vi "读取校准数据.vi"(8 "error in (no error)":errorcluster) -> (0 "error out":errorcluster)   [LabVIEW 2016, in "斯坦道通用流路CODmn.lvlib"]
uses:
  <vilib>/Utility/config.llb/NI_LVConfig.lvlib
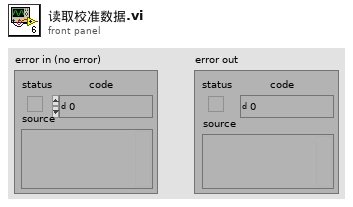
[diagram p1: front panel]
types:
  T1 = cluster{"参数":cluster{"String":string, "Value":u16}, "曲线模型":cluster{"标液浓度1":dbl, "测量吸光度1":dbl, "样品1启用":bool, "标液浓度2":dbl, "测量吸光度2":dbl, "样品2启用":bool, "标液浓度3":dbl, "测量吸光度3":dbl, "样品3启用":bool, "标液浓度4":dbl, "测量吸光度4":dbl, "样品4启用":bool, "标液浓度5":dbl, "测量吸光度5":dbl, "样品5启用":bool, "模型":enum32{"线性", "多项式"}, "精度":dbl, "XY图":cluster{"X Values":dbl[], "Y Values":dbl[]}[], "拟合公式":string, "r^2":dbl, "标样一校准时间":timestamp, "标样二校准时间":timestamp, "标样三校准时间":timestamp, "标样四校准时间":timestamp, "标样五校准时间":timestamp, "方程":cluster{"c":dbl, "x":dbl, "x^2":dbl}, "标定时间":timestamp}[]}[]
  T2 = cluster{"标液浓度1":dbl, "测量吸光度1":dbl, "样品1启用":bool, "标液浓度2":dbl, "测量吸光度2":dbl, "样品2启用":bool, "标液浓度3":dbl, "测量吸光度3":dbl, "样品3启用":bool, "标液浓度4":dbl, "测量吸光度4":dbl, "样品4启用":bool, "标液浓度5":dbl, "测量吸光度5":dbl, "样品5启用":bool, "模型":enum32{"线性", "多项式"}, "精度":dbl, "XY图":cluster{"X Values":dbl[], "Y Values":dbl[]}[], "拟合公式":string, "r^2":dbl, "标样一校准时间":timestamp, "标样二校准时间":timestamp, "标样三校准时间":timestamp, "标样四校准时间":timestamp, "标样五校准时间":timestamp, "二次方程":cluster{"c":dbl, "x":dbl, "x^2":dbl}, "标定时间":timestamp}[]
  T3 = cluster{cluster{"String":string, "Value":u16}, "总磷曲线模型":cluster{"标液浓度1":dbl, "测量吸光度1":dbl, "样品1启用":bool, "标液浓度2":dbl, "测量吸光度2":dbl, "样品2启用":bool, "标液浓度3":dbl, "测量吸光度3":dbl, "样品3启用":bool, "标液浓度4":dbl, "测量吸光度4":dbl, "样品4启用":bool, "标液浓度5":dbl, "测量吸光度5":dbl, "样品5启用":bool, "模型":enum32{"线性", "多项式"}, "精度":dbl, "XY图":cluster{"X Values":dbl[], "Y Values":dbl[]}[], "拟合公式":string, "r^2":dbl, "标样一校准时间":timestamp, "标样二校准时间":timestamp, "标样三校准时间":timestamp, "标样四校准时间":timestamp, "标样五校准时间":timestamp, "二次方程":cluster{"c":dbl, "x":dbl, "x^2":dbl}, "标定时间":timestamp}[]}
  T4 = cluster{cluster{"String":string, "Value":u16}, "总氮曲线模型":cluster{"标液浓度1":dbl, "测量吸光度1":dbl, "样品1启用":bool, "标液浓度2":dbl, "测量吸光度2":dbl, "样品2启用":bool, "标液浓度3":dbl, "测量吸光度3":dbl, "样品3启用":bool, "标液浓度4":dbl, "测量吸光度4":dbl, "样品4启用":bool, "标液浓度5":dbl, "测量吸光度5":dbl, "样品5启用":bool, "模型":enum32{"线性", "多项式"}, "精度":dbl, "XY图":cluster{"X Values":dbl[], "Y Values":dbl[]}[], "拟合公式":string, "r^2":dbl, "标样一校准时间":timestamp, "标样二校准时间":timestamp, "标样三校准时间":timestamp, "标样四校准时间":timestamp, "标样五校准时间":timestamp, "二次方程":cluster{"c":dbl, "x":dbl, "x^2":dbl}, "标定时间":timestamp}[]}
  T5 = cluster{cluster{"String":string, "Value":u16}, "氨氮曲线模型":cluster{"标液浓度1":dbl, "测量吸光度1":dbl, "样品1启用":bool, "标液浓度2":dbl, "测量吸光度2":dbl, "样品2启用":bool, "标液浓度3":dbl, "测量吸光度3":dbl, "样品3启用":bool, "标液浓度4":dbl, "测量吸光度4":dbl, "样品4启用":bool, "标液浓度5":dbl, "测量吸光度5":dbl, "样品5启用":bool, "模型":enum32{"线性", "多项式"}, "精度":dbl, "XY图":cluster{"X Values":dbl[], "Y Values":dbl[]}[], "拟合公式":string, "r^2":dbl, "标样一校准时间":timestamp, "标样二校准时间":timestamp, "标样三校准时间":timestamp, "标样四校准时间":timestamp, "标样五校准时间":timestamp, "二次方程":cluster{"c":dbl, "x":dbl, "x^2":dbl}, "标定时间":timestamp}[]}
  T6 = cluster{cluster{"String":string, "Value":u16}, "磷酸盐曲线模型":cluster{"标液浓度1":dbl, "测量吸光度1":dbl, "样品1启用":bool, "标液浓度2":dbl, "测量吸光度2":dbl, "样品2启用":bool, "标液浓度3":dbl, "测量吸光度3":dbl, "样品3启用":bool, "标液浓度4":dbl, "测量吸光度4":dbl, "样品4启用":bool, "标液浓度5":dbl, "测量吸光度5":dbl, "样品5启用":bool, "模型":enum32{"线性", "多项式"}, "精度":dbl, "XY图":cluster{"X Values":dbl[], "Y Values":dbl[]}[], "拟合公式":string, "r^2":dbl, "标样一校准时间":timestamp, "标样二校准时间":timestamp, "标样三校准时间":timestamp, "标样四校准时间":timestamp, "标样五校准时间":timestamp, "二次方程":cluster{"c":dbl, "x":dbl, "x^2":dbl}, "标定时间":timestamp}[]}
  T7 = cluster{cluster{"String":string, "Value":u16}, "硝氮曲线模型":cluster{"标液浓度1":dbl, "测量吸光度1":dbl, "样品1启用":bool, "标液浓度2":dbl, "测量吸光度2":dbl, "样品2启用":bool, "标液浓度3":dbl, "测量吸光度3":dbl, "样品3启用":bool, "标液浓度4":dbl, "测量吸光度4":dbl, "样品4启用":bool, "标液浓度5":dbl, "测量吸光度5":dbl, "样品5启用":bool, "模型":enum32{"线性", "多项式"}, "精度":dbl, "XY图":cluster{"X Values":dbl[], "Y Values":dbl[]}[], "拟合公式":string, "r^2":dbl, "标样一校准时间":timestamp, "标样二校准时间":timestamp, "标样三校准时间":timestamp, "标样四校准时间":timestamp, "标样五校准时间":timestamp, "二次方程":cluster{"c":dbl, "x":dbl, "x^2":dbl}, "标定时间":timestamp}[]}
  T8 = cluster{cluster{"String":string, "Value":u16}, "亚硝氮曲线模型":cluster{"标液浓度1":dbl, "测量吸光度1":dbl, "样品1启用":bool, "标液浓度2":dbl, "测量吸光度2":dbl, "样品2启用":bool, "标液浓度3":dbl, "测量吸光度3":dbl, "样品3启用":bool, "标液浓度4":dbl, "测量吸光度4":dbl, "样品4启用":bool, "标液浓度5":dbl, "测量吸光度5":dbl, "样品5启用":bool, "模型":enum32{"线性", "多项式"}, "精度":dbl, "XY图":cluster{"X Values":dbl[], "Y Values":dbl[]}[], "拟合公式":string, "r^2":dbl, "标样一校准时间":timestamp, "标样二校准时间":timestamp, "标样三校准时间":timestamp, "标样四校准时间":timestamp, "标样五校准时间":timestamp, "二次方程":cluster{"c":dbl, "x":dbl, "x^2":dbl}, "标定时间":timestamp}[]}
  T9 = cluster{cluster{"String":string, "Value":u16}, "硅酸盐曲线模型":cluster{"标液浓度1":dbl, "测量吸光度1":dbl, "样品1启用":bool, "标液浓度2":dbl, "测量吸光度2":dbl, "样品2启用":bool, "标液浓度3":dbl, "测量吸光度3":dbl, "样品3启用":bool, "标液浓度4":dbl, "测量吸光度4":dbl, "样品4启用":bool, "标液浓度5":dbl, "测量吸光度5":dbl, "样品5启用":bool, "模型":enum32{"线性", "多项式"}, "精度":dbl, "XY图":cluster{"X Values":dbl[], "Y Values":dbl[]}[], "拟合公式":string, "r^2":dbl, "标样一校准时间":timestamp, "标样二校准时间":timestamp, "标样三校准时间":timestamp, "标样四校准时间":timestamp, "标样五校准时间":timestamp, "二次方程":cluster{"c":dbl, "x":dbl, "x^2":dbl}, "标定时间":timestamp}[]}
  T10 = cluster{cluster{"String":string, "Value":u16}, "硫化物曲线模型":cluster{"标液浓度1":dbl, "测量吸光度1":dbl, "样品1启用":bool, "标液浓度2":dbl, "测量吸光度2":dbl, "样品2启用":bool, "标液浓度3":dbl, "测量吸光度3":dbl, "样品3启用":bool, "标液浓度4":dbl, "测量吸光度4":dbl, "样品4启用":bool, "标液浓度5":dbl, "测量吸光度5":dbl, "样品5启用":bool, "模型":enum32{"线性", "多项式"}, "精度":dbl, "XY图":cluster{"X Values":dbl[], "Y Values":dbl[]}[], "拟合公式":string, "r^2":dbl, "标样一校准时间":timestamp, "标样二校准时间":timestamp, "标样三校准时间":timestamp, "标样四校准时间":timestamp, "标样五校准时间":timestamp, "二次方程":cluster{"c":dbl, "x":dbl, "x^2":dbl}, "标定时间":timestamp}[]}
  T11 = cluster{cluster{"String":string, "Value":u16}, "CODcr曲线模型":cluster{"标液浓度1":dbl, "测量吸光度1":dbl, "样品1启用":bool, "标液浓度2":dbl, "测量吸光度2":dbl, "样品2启用":bool, "标液浓度3":dbl, "测量吸光度3":dbl, "样品3启用":bool, "标液浓度4":dbl, "测量吸光度4":dbl, "样品4启用":bool, "标液浓度5":dbl, "测量吸光度5":dbl, "样品5启用":bool, "模型":enum32{"线性", "多项式"}, "精度":dbl, "XY图":cluster{"X Values":dbl[], "Y Values":dbl[]}[], "拟合公式":string, "r^2":dbl, "标样一校准时间":timestamp, "标样二校准时间":timestamp, "标样三校准时间":timestamp, "标样四校准时间":timestamp, "标样五校准时间":timestamp, "二次方程":cluster{"c":dbl, "x":dbl, "x^2":dbl}, "标定时间":timestamp}[]}
  T12 = cluster{cluster{"String":string, "Value":u16}, "CODMn曲线模型":cluster{"标液浓度1":dbl, "测量吸光度1":dbl, "样品1启用":bool, "标液浓度2":dbl, "测量吸光度2":dbl, "样品2启用":bool, "标液浓度3":dbl, "测量吸光度3":dbl, "样品3启用":bool, "标液浓度4":dbl, "测量吸光度4":dbl, "样品4启用":bool, "标液浓度5":dbl, "测量吸光度5":dbl, "样品5启用":bool, "模型":enum32{"线性", "多项式"}, "精度":dbl, "XY图":cluster{"X Values":dbl[], "Y Values":dbl[]}[], "拟合公式":string, "r^2":dbl, "标样一校准时间":timestamp, "标样二校准时间":timestamp, "标样三校准时间":timestamp, "标样四校准时间":timestamp, "标样五校准时间":timestamp, "二次方程":cluster{"c":dbl, "x":dbl, "x^2":dbl}, "标定时间":timestamp}[]}
  T13 = cluster{cluster{"String":string, "Value":u16}, "氟化物曲线模型":cluster{"标液浓度1":dbl, "测量吸光度1":dbl, "样品1启用":bool, "标液浓度2":dbl, "测量吸光度2":dbl, "样品2启用":bool, "标液浓度3":dbl, "测量吸光度3":dbl, "样品3启用":bool, "标液浓度4":dbl, "测量吸光度4":dbl, "样品4启用":bool, "标液浓度5":dbl, "测量吸光度5":dbl, "样品5启用":bool, "模型":enum32{"线性", "多项式"}, "精度":dbl, "XY图":cluster{"X Values":dbl[], "Y Values":dbl[]}[], "拟合公式":string, "r^2":dbl, "标样一校准时间":timestamp, "标样二校准时间":timestamp, "标样三校准时间":timestamp, "标样四校准时间":timestamp, "标样五校准时间":timestamp, "二次方程":cluster{"c":dbl, "x":dbl, "x^2":dbl}, "标定时间":timestamp}[]}
  T14 = typedef "NI_LVConfig.lvlib/Config Data RefNum.ctl" = refnum<k1>
  T15 = cluster{"参数":cluster{"String":string, "Value":u16}, "曲线模型":cluster{"标液浓度1":dbl, "测量吸光度1":dbl, "样品1启用":bool, "标液浓度2":dbl, "测量吸光度2":dbl, "样品2启用":bool, "标液浓度3":dbl, "测量吸光度3":dbl, "样品3启用":bool, "标液浓度4":dbl, "测量吸光度4":dbl, "样品4启用":bool, "标液浓度5":dbl, "测量吸光度5":dbl, "样品5启用":bool, "模型":enum32{"线性", "多项式"}, "精度":dbl, "XY图":cluster{"X Values":dbl[], "Y Values":dbl[]}[], "拟合公式":string, "r^2":dbl, "标样一校准时间":timestamp, "标样二校准时间":timestamp, "标样三校准时间":timestamp, "标样四校准时间":timestamp, "标样五校准时间":timestamp, "方程":cluster{"c":dbl, "x":dbl, "x^2":dbl}, "标定时间":timestamp}[]}
  T16 = cluster{"标液浓度1":dbl, "测量吸光度1":dbl, "样品1启用":bool, "标液浓度2":dbl, "测量吸光度2":dbl, "样品2启用":bool, "标液浓度3":dbl, "测量吸光度3":dbl, "样品3启用":bool, "标液浓度4":dbl, "测量吸光度4":dbl, "样品4启用":bool, "标液浓度5":dbl, "测量吸光度5":dbl, "样品5启用":bool, "模型":enum32{"线性", "多项式"}, "精度":dbl, "XY图":cluster{"X Values":dbl[], "Y Values":dbl[]}[], "拟合公式":string, "r^2":dbl, "标样一校准时间":timestamp, "标样二校准时间":timestamp, "标样三校准时间":timestamp, "标样四校准时间":timestamp, "标样五校准时间":timestamp, "方程":cluster{"c":dbl, "x":dbl, "x^2":dbl}, "标定时间":timestamp}[]
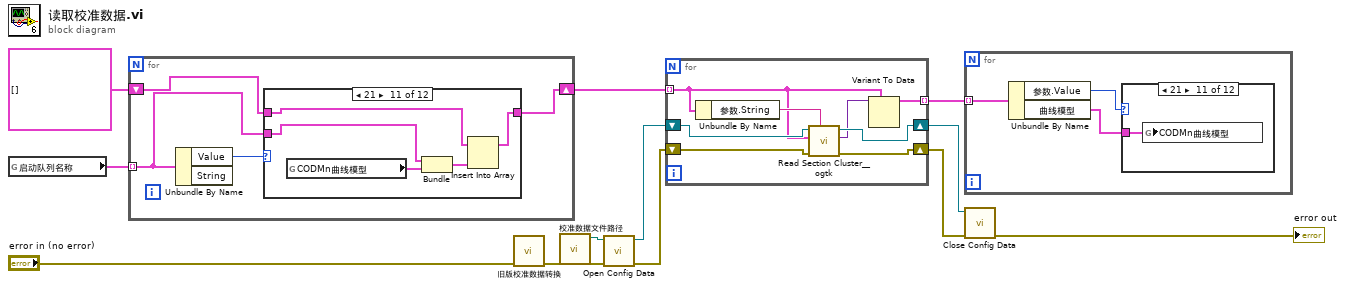
[diagram p0: block diagram]
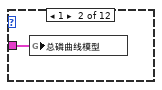
[diagram p3: hidden frame]
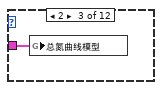
[diagram p4: hidden frame]
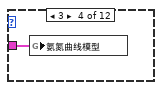
[diagram p5: hidden frame]
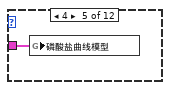
[diagram p6: hidden frame]
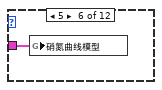
[diagram p7: hidden frame]
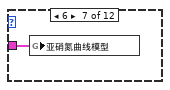
[diagram p8: hidden frame]
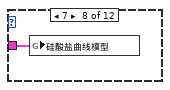
[diagram p9: hidden frame]
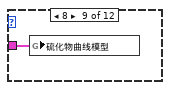
[diagram p10: hidden frame]
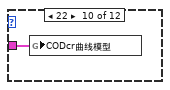
[diagram p11: hidden frame]
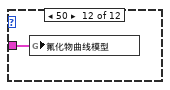
[diagram p12: hidden frame]
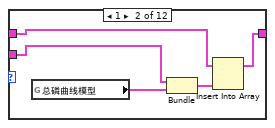
[diagram p14: hidden frame]
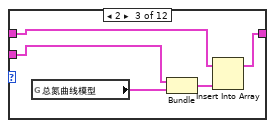
[diagram p15: hidden frame]
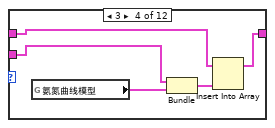
[diagram p16: hidden frame]
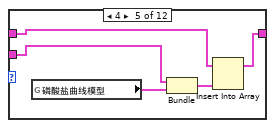
[diagram p17: hidden frame]
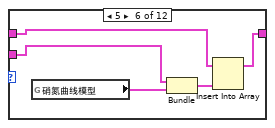
[diagram p18: hidden frame]
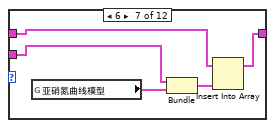
[diagram p19: hidden frame]
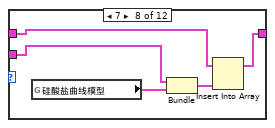
[diagram p20: hidden frame]
diagram:
  n1 = global read "model config var.vi" "启动队列名称"() -> (w12:cluster{"String":string, "Value":u16}[])
  n2 = for {
    tunnel: w12 -> [w13] mode=indexing
    shift-right: [w15] -> w6
    shift-left: T1 [] ("曲线模型") -> [w14]
    n3 = Unbundle By Name(w13) -> ("Value"=w16:u16)  [unwired: 1 out]
    n4 = case shown="21" w16 {
      tunnel: [w17 w21 w26 w31 w36 w41 w46 w51 w56 w61 w66 w71] -> w15
      tunnel: w14 -> [w17 w22 w27 w32 w37 w42 w47 w52 w57 w62 w67 w72]
      tunnel: w13 -> [_ w19 w23 w29 w34 w39 w44 w49 w54 w59 w64 w69]
      frame 0, Default {
      }
      frame 1 {
        n5 = global read "校准数据全局变量.vi" "总磷曲线模型"() -> (w20:T2)
        n6 = Bundle(w19, "总磷曲线模型"=w20) -> (w18:T3)  [unwired: 1 in]
        n7 = Insert Into Array(array=w22, new element=w18) -> (w21:T1)  [unwired: 1 in]
      }
      frame 2 {
        n8 = global read "校准数据全局变量.vi" "总氮曲线模型"() -> (w25:T2)
        n9 = Bundle(w23, "总氮曲线模型"=w25) -> (w24:T4)  [unwired: 1 in]
        n10 = Insert Into Array(array=w27, new element=w24) -> (w26:T1)  [unwired: 1 in]
      }
      frame 3 {
        n11 = global read "校准数据全局变量.vi" "氨氮曲线模型"() -> (w30:T2)
        n12 = Bundle(w29, "氨氮曲线模型"=w30) -> (w28:T5)  [unwired: 1 in]
        n13 = Insert Into Array(array=w32, new element=w28) -> (w31:T1)  [unwired: 1 in]
      }
      frame 4 {
        n14 = global read "校准数据全局变量.vi" "磷酸盐曲线模型"() -> (w35:T2)
        n15 = Bundle(w34, "磷酸盐曲线模型"=w35) -> (w33:T6)  [unwired: 1 in]
        n16 = Insert Into Array(array=w37, new element=w33) -> (w36:T1)  [unwired: 1 in]
      }
      frame 5 {
        n17 = global read "校准数据全局变量.vi" "硝氮曲线模型"() -> (w40:T2)
        n18 = Bundle(w39, "硝氮曲线模型"=w40) -> (w38:T7)  [unwired: 1 in]
        n19 = Insert Into Array(array=w42, new element=w38) -> (w41:T1)  [unwired: 1 in]
      }
      frame 6 {
        n20 = global read "校准数据全局变量.vi" "亚硝氮曲线模型"() -> (w45:T2)
        n21 = Bundle(w44, "亚硝氮曲线模型"=w45) -> (w43:T8)  [unwired: 1 in]
        n22 = Insert Into Array(array=w47, new element=w43) -> (w46:T1)  [unwired: 1 in]
      }
      frame 7 {
        n23 = global read "校准数据全局变量.vi" "硅酸盐曲线模型"() -> (w50:T2)
        n24 = Bundle(w49, "硅酸盐曲线模型"=w50) -> (w48:T9)  [unwired: 1 in]
        n25 = Insert Into Array(array=w52, new element=w48) -> (w51:T1)  [unwired: 1 in]
      }
      frame 8 {
        n26 = global read "校准数据全局变量.vi" "硫化物曲线模型"() -> (w55:T2)
        n27 = Bundle(w54, "硫化物曲线模型"=w55) -> (w53:T10)  [unwired: 1 in]
        n28 = Insert Into Array(array=w57, new element=w53) -> (w56:T1)  [unwired: 1 in]
      }
      frame 22 {
        n29 = global read "校准数据全局变量.vi" "CODcr曲线模型"() -> (w60:T2)
        n30 = Bundle(w59, "CODcr曲线模型"=w60) -> (w58:T11)  [unwired: 1 in]
        n31 = Insert Into Array(array=w62, new element=w58) -> (w61:T1)  [unwired: 1 in]
      }
      frame 21 {
        n32 = global read "校准数据全局变量.vi" "CODMn曲线模型"() -> (w65:T2)
        n33 = Bundle(w64, "CODMn曲线模型"=w65) -> (w63:T12)  [unwired: 1 in]
        n34 = Insert Into Array(array=w67, new element=w63) -> (w66:T1)  [unwired: 1 in]
      }
      frame 50 {
        n35 = global read "校准数据全局变量.vi" "氟化物曲线模型"() -> (w70:T2)
        n36 = Bundle(w69, "氟化物曲线模型"=w70) -> (w68:T13)  [unwired: 1 in]
        n37 = Insert Into Array(array=w72, new element=w68) -> (w71:T1)  [unwired: 1 in]
      }
    }
  }
  n38 = call "旧版校准数据转换.vi"("error in (no error)"="error in (no error)") -> ("error out"=w5:errorcluster)  [unwired: 10 in]
  n39 = call "校准数据文件路径.vi"() -> ("appended path"=w1:path)  [unwired: 11 in]
  n40 = call <vilib>:"Open Config Data.vi"("error in (no error)"=w5, "configuration file path"=w1) -> ("error out"=w10:errorcluster, "refnum"=w9:T14)  [unwired: 7 in, 1 out]
  n41 = for {
    shift-right: [w77] -> w7
    shift-left: w10 -> [w80]
    shift-right: [w78] -> w8
    shift-left: w9 -> [w79]
    tunnel: w6 -> [w74] mode=indexing
    tunnel: [w73] -> w2 mode=indexing
    n42 = Unbundle By Name(w74) -> ("参数.String"=w76:string)
    n43 = call <userlib>:"Read Section Cluster__ogtk.vi"("section (optional)"=w76, "error in (no error)"=w80, "Section Formatted Cluster Type"=w74, "refnum"=w79) -> ("error out"=w77:errorcluster, "Section Formatted Cluster"=w75:variant, "dup refnum"=w78:T14)  [unwired: 3 in, 2 out]
    n44 = Variant To Data(type=w74, Variant=w75) -> (data=w73:T15)  [unwired: 1 in, 1 out]
  }
  n45 = for {
    tunnel: w2 -> [w83] mode=indexing
    n46 = Unbundle By Name(w83) -> ("参数.Value"=w82:u16, "曲线模型"=w81:T16)
    n47 = case shown="21" w82 {
      tunnel: w81 -> [_ w84 w85 w86 w87 w88 w89 w90 w91 w92 w93 w94]
      frame 0, Default {
      }
      frame 1 {
        n48 = global write "校准数据全局变量.vi" "总磷曲线模型"(w84) -> ()
      }
      frame 2 {
        n49 = global write "校准数据全局变量.vi" "总氮曲线模型"(w85) -> ()
      }
      frame 3 {
        n50 = global write "校准数据全局变量.vi" "氨氮曲线模型"(w86) -> ()
      }
      frame 4 {
        n51 = global write "校准数据全局变量.vi" "磷酸盐曲线模型"(w87) -> ()
      }
      frame 5 {
        n52 = global write "校准数据全局变量.vi" "硝氮曲线模型"(w88) -> ()
      }
      frame 6 {
        n53 = global write "校准数据全局变量.vi" "亚硝氮曲线模型"(w89) -> ()
      }
      frame 7 {
        n54 = global write "校准数据全局变量.vi" "硅酸盐曲线模型"(w90) -> ()
      }
      frame 8 {
        n55 = global write "校准数据全局变量.vi" "硫化物曲线模型"(w91) -> ()
      }
      frame 22 {
        n56 = global write "校准数据全局变量.vi" "CODcr曲线模型"(w92) -> ()
      }
      frame 21 {
        n57 = global write "校准数据全局变量.vi" "CODMn曲线模型"(w93) -> ()
      }
      frame 50 {
        n58 = global write "校准数据全局变量.vi" "氟化物曲线模型"(w94) -> ()
      }
    }
  }
  n59 = call <vilib>:"Close Config Data.vi"("error in (no error)"=w7, "refnum"=w8) -> ("error out"=→"error out":errorcluster)  [unwired: 8 in, 1 out]
